vi "MH_UDP Multicast Receiver.vi"() -> ()   [LabVIEW 2010]
doc: "Demonstrates how to work with the UDP Multicast Sender.vi. Run this VI first.\n\nUDP multicast will allow LabVIEW to send data to a multicast group or to receive data sent to a multicast group. In LabVIEW, UDP multicast is used in very much the same way as UDP. The main difference is there are two new parameters, TTL and Multicast Address, on the UDP Multicast Open. \n\nWhen sending to a multicast group the default time-to-live (TTL) is 1, which only allows the packet to go to the local subnet. When a router receives a multicast packet, it decrements the packets TTL, and if the TTL is greater than 0, forwards the packet to other routers.\nA multicast group is defined by having a multicast IP address in the range 224.0.0.0 to 239.255.255.255."
uses:
  <vilib>/Utility/tcp.llb/UDP Multicast Open.vi
panel:
  out "freq.":dbl
  in  "stop":bool
  in  "Multicast Address":string="234.5.6.7"
  in  "Port":i32=58432
  out "Data Received":string
  # "Instructions:\n1. Open the UDP Multicast Sender.vi located in the same library.\n2. Make sure that Port in this VI and Send to Port in the UDP Multicast Sender.vi are the same and that they have the same Multicast Address.\n3. Run this VI first\n4. Run the UDP Multicast Sender VI second\nNote: This VI is built to work with the UDP Multicast Sender.vi."
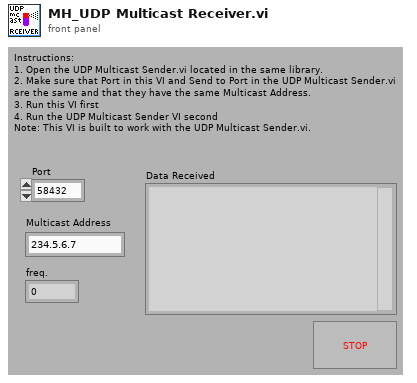
[diagram p1: front panel]
types:
  T1 = typedef "IMAQ Image.ctl" = refnum<image>
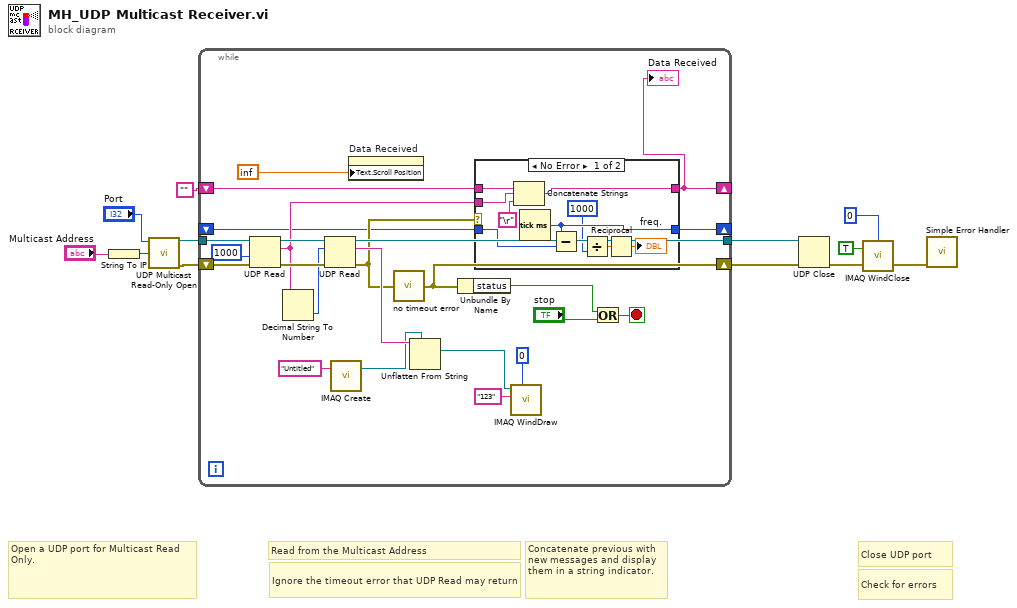
[diagram p0: block diagram]
diagram:
  # "Open a UDP port for Multicast Read Only."
  # "Read from the Multicast Address"
  # "Close UDP port"
  # "Check for errors"
  # "Concatenate previous with new messages and display them in a string indicator."
  # "Ignore the timeout error that UDP Read may return"
  n1 = String To IP(1:"Multicast Address") -> (0:w9:u32)
  n2 = call-poly <vilib>:"UDP Multicast Read-Only Open.vi"("multicast addr"=w9, "port"="Port") -> ("error out"=w10:errorcluster, "connection ID"=w12:refnum<k16>)  [unwired: 2 in, 6 out]
  n3 = while {
    tunnel: w12 -> [w36]
    tunnel: [w27] -> w11
    shift-right: [w34] -> _
    shift-left: "" -> [w35]
    shift-right: [w15] -> w5
    shift-left: w10 -> [w30]
    shift-right: [w14] -> _
    shift-left: _ -> [w13]
    stop <- w32 stop-if-true
    n4 = UDP Read(connection ID=w36, timeout ms (25000)=1000, 8:w30) -> (data out=w25:string, error out=w26:errorcluster, 3:w28:refnum<k16>)  [unwired: 3 out]
    n5 = Decimal String To Number(string=w25) -> (number=w24:i32)  [unwired: 2 in, 1 out]
    n6 = UDP Read(connection ID=w28, max size (548)=w24, 8:w26) -> (data out=w23:string, error out=w16:errorcluster, 3:w27:refnum<k16>)  [unwired: 1 in, 2 out]
    n7 = call "IMAQ Create"("Image Name"="Untitled") -> ("New Image"=w21:T1)  [unwired: 4 in, 1 out]
    n8 = property on="Data Received" class="Str"("Text.Scroll Position"=inf) -> ()  [unwired: 2 in, 2 out]
    n9 = call "no timeout error.vi"("error in (no error)"=w16) -> ("error out"=w15:errorcluster)
    n10 = Unflatten From String(type=w21, binary string=w23) -> (value=w18:T1)  [unwired: 3 in, 2 out]
    n11 = Unbundle By Name(w15) -> ("status"=w17:bool)
    n12 = case shown="No Error" w16 {
      tunnel: w35 -> [w46 w48]
      tunnel: w25 -> [w44 _]
      tunnel: [w45 w48] -> w34
      tunnel: [w42 w47] -> w14
      tunnel: w13 -> [w41 w47]
      frame No Error {
        n13 = Concatenate Strings(w46, w44, "\r") -> (w45:string)
        n14 = Tick Count (ms)() -> (millisecond timer value=w42:u32)
        n15 = Subtract(x=w42, y=w41) -> (x-y=w39:u32)
        n16 = Divide(x=w39, y=u32 1000) -> (x/y=w37:dbl)
        n17 = Reciprocal(x=w37) -> (1/x=→"freq.":dbl)
      }
      frame Error {
      }
    }
    "Data Received" <- w34
    n18 = call "IMAQ WindDraw"("Window Number (0...15)"=0, "Title"="123", "Image"=w18) -> ()  [unwired: 7 in, 2 out]
    n19 = Or(x=w17, y="stop") -> (x .or. y?=w32:bool)
  }
  n20 = UDP Close(connection ID=w11, 8:w5) -> (error out=w2:errorcluster)  [unwired: 1 out]
  n21 = call "IMAQ WindClose"("Window Number (0...15)"=0, "Close All Windows (False)"=TRUE, "error in (no error)"=w2) -> ("error out"=w1:errorcluster)  [unwired: 3 in]
  n22 = call <vilib>:"Simple Error Handler.vi"("error in (no error)"=w1) -> ()  [unwired: 1 in, 8 out]
